vi "SR400 GetCountSource.vi"(7 "error in (no error)":errorcluster, 10 "VISA Port In":refnum<visa-resource-name>="GPIB0::23::INSTR") -> (0 "error out":errorcluster, 1 "T Source":u16(ring) caption="Source «T»" items=["10 MHz"=0, "Input 2"=2, "Trig"=3], 2 "B Source":u16(ring)=2 caption="Source «B»" items=["Input 1"=1, "Input 2"=2], 3 "VISA Port Out":refnum<visa-resource-name>="GPIB0::23::INSTR", 4 "A Source":u16(ring)=1 caption="Source «A»" items=["Input 1"=1, "10 MHz"=0])   [LabVIEW 2019]
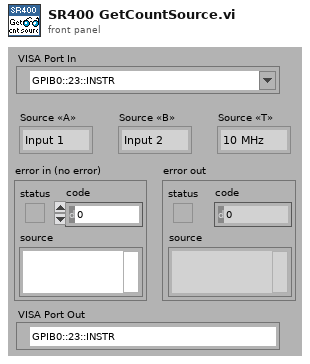
[diagram p1: front panel]
types:
  T1 = enum16{"Lit le Statut", "Demande Param", "Lit Param", "Oper. incomp."}
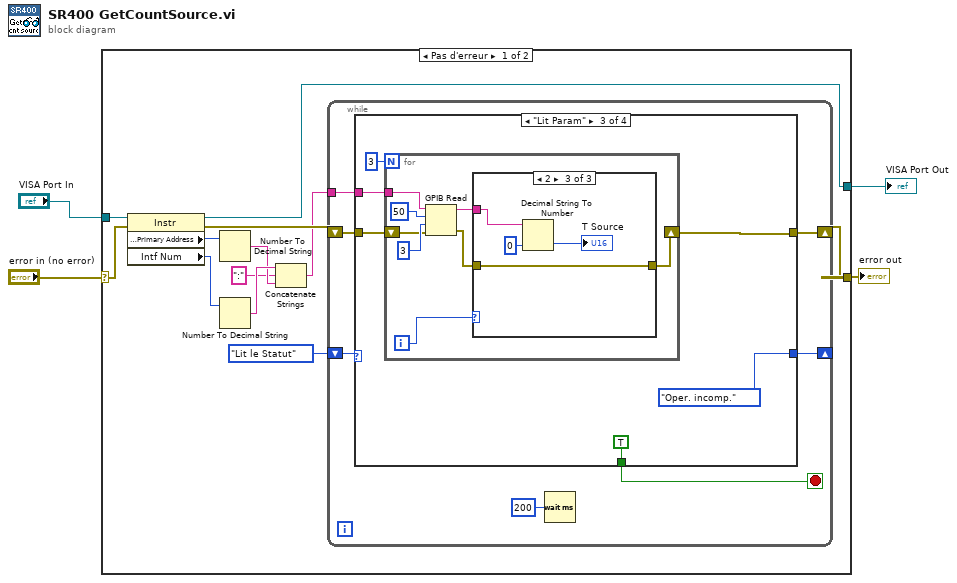
[diagram p0: block diagram]
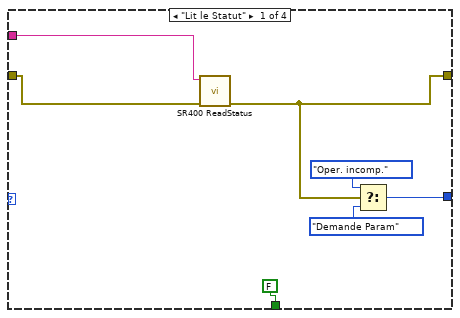
[diagram p2: hidden frame]
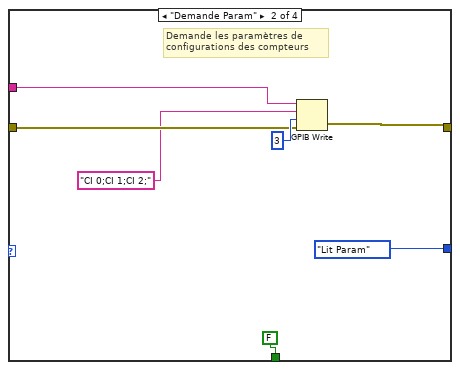
[diagram p3: hidden frame]
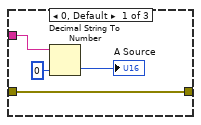
[diagram p4: hidden frame]
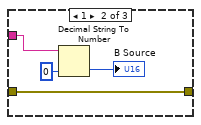
[diagram p5: hidden frame]
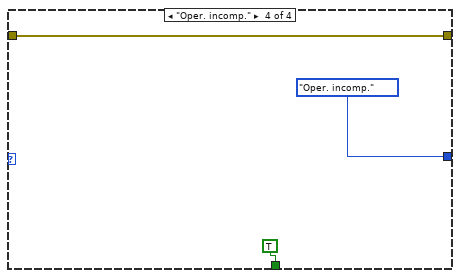
[diagram p6: hidden frame]
diagram:
  n1 = case shown="Pas d'erreur" "error in (no error)" {
    selector: "error in (no error)" -> [w16 w68]
    tunnel: [w12 w68] -> w3
    tunnel: "VISA Port In" -> [w15 w67]
    tunnel: [w6 w67] -> w1
    frame No Error {
      n2 = property class="Instr"(reference=w15, error in=w16) -> (reference out=w6:refnum<visa-resource-name>, error out=w14:errorcluster, "GPIB Settings:Primary Address"=w13:u16, "Intf Num"=w5:u16)
      n3 = Number To Decimal String(number=w13) -> (decimal integer string=w9:string)  [unwired: 1 in]
      n4 = Number To Decimal String(number=w5) -> (decimal integer string=w10:string)  [unwired: 1 in]
      n5 = Concatenate Strings(w10, ":" ("string"), w9) -> (w7:string)
      n6 = while {
        shift-right: [w18] -> _
        shift-left: T1."Lit le Statut" -> [w23]
        tunnel: w7 -> [w21]
        shift-right: [w20] -> w12
        shift-left: w14 -> [w22]
        stop <- w19 stop-if-true
        n7 = case shown="\"Lit Param\"" w23 {
          tunnel: w22 -> [w29 w35 w41 w66]
          tunnel: w21 -> [w28 w34 w40 _]
          tunnel: [w24 w31 w38 w66] -> w20
          tunnel: [FALSE ("Configuration\neffectuée") FALSE ("Configuration\neffectuée") TRUE ("Configuration\neffectuée") TRUE ("Configuration\neffectuée")] -> w19
          tunnel: [w27 T1."Lit Param" T1."Oper. incomp." T1."Oper. incomp."] -> w18
          frame "Lit le Statut" {
            n8 = call <userlib>:"SR400 ReadStatus.vi"("error in"=w29, "Address string"=w28) -> ("Error Out"=w24:errorcluster)  [unwired: 6 in, 1 out]
            n9 = Select(t=T1."Oper. incomp.", s=w24, f=T1."Demande Param") -> (s? t:f=w27:T1)
          }
          frame "Demande Param" {
            # "Demande les paramètres de configurations des compteurs"
            n10 = GPIB Write(0:w34, 1:"CI 0;CI 1;CI 2;", 2:i16 3 ("mode (0)"), 3:w35) -> (6:w31:errorcluster)  [unwired: 1 in, 1 out]
          }
          frame "Lit Param" {
            n11 = for {
              N: 3 -> [_]
              shift-right: [w44] -> w38
              shift-left: w41 -> [w48]
              tunnel: w40 -> [w49]
              i -> [w47]
              n12 = GPIB Read(0:w49, 1:50 ("byte count"), 2:i16 3 ("mode (0)"), 3:w48) -> (5:w45:string, 7:w46:errorcluster)  [unwired: 1 in, 1 out]
              n13 = case shown="2" w47 {
                tunnel: w46 -> [w52 w59 w63]
                tunnel: w45 -> [w54 w57 w61]
                tunnel: [w52 w59 w63] -> w44
                frame 0, Default {
                  n14 = Decimal String To Number(string=w54, default (0L)=u16 0 ("default (0 I32)")) -> (number=→"A Source":u16)  [unwired: 1 in, 1 out]
                }
                frame 1 {
                  n15 = Decimal String To Number(string=w57, default (0L)=u16 0 ("default (0 I32)")) -> (number=→"B Source":u16)  [unwired: 1 in, 1 out]
                }
                frame 2 {
                  n16 = Decimal String To Number(string=w61, default (0L)=u16 0 ("default (0 I32)")) -> (number=→"T Source":u16)  [unwired: 1 in, 1 out]
                }
              }
            }
          }
          frame "Oper. incomp." {
          }
        }
        n17 = Wait (ms)(milliseconds to wait=u32 200) -> ()  [unwired: 1 out]
      }
    }
    frame Error {
    }
  }
  "error out" <- w3
  "VISA Port Out" <- w1
